vi "HostCurrentSampling.vi"() -> ()   [LabVIEW 2014]
uses:
  <vilib>/FPGAPlugInAG/PCIe-7851R/niLvFpga_Open_PCIe-7851R.vi
  <vilib>/rvi/interface/common/dynamic/niFpgaDynamicAddResources.vi
  <vilib>/Utility/error.llb/Error Cluster From Error Code.vi
  <vilib>/rvi/errors/niLvFpgaAdjustHostInterfaceError.vi
  <vilib>/FPGAPlugInAG/Dynamic/niLvFpga_Close_Dynamic.vi
  <vilib>/rvi/interface/nirviOpenFPGA/nirviOpenFPGA.xnode
  FPGA Bitfiles/UntitledProject1_FPGATarget_FPGACurrentSampl_waaLAvbA01k.lvbitx
  <vilib>/rvi/interface/nirviReadWriteControl/nirviReadWriteControl.xnode
  <vilib>/rvi/interface/nirviMethod/nirviMethod.xnode
  <vilib>/rvi/interface/nirviCloseFPGA/nirviCloseFPGA.xnode
  NiFpgaLv.dll
  <vilib>/rvi/interface/Simulation/niFpgaSimulationCallBeginRW.vi
  <vilib>/FPGAPlugInAG/Dynamic/niLvFpga_ReadFifo_Dynamic.vi
  <vilib>/rvi/errors/niLvFpgaMergeErrorWithErrorCode.vi
panel:
  in  "Count(uSec)":u32
  out "PresNum":i32
  in  "SampleNum":i32
  in  "stop":bool
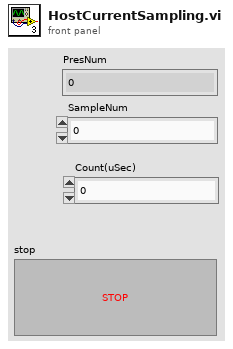
[diagram p1: front panel]
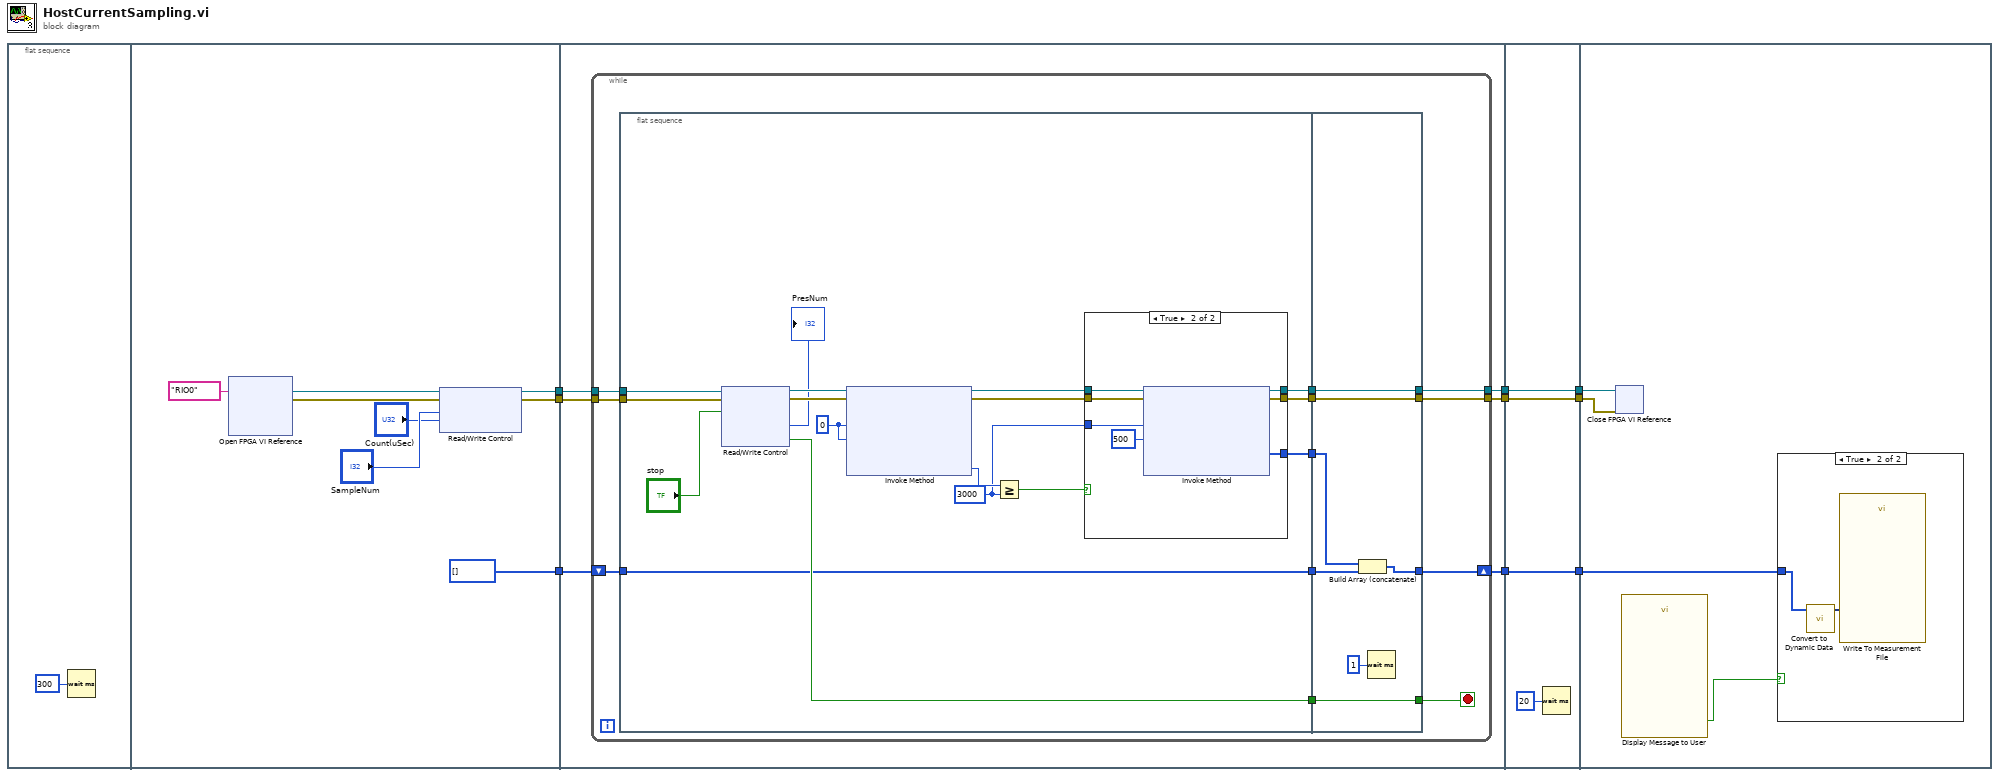
[diagram p0: block diagram]
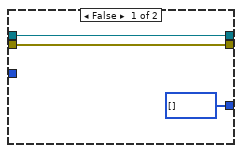
[diagram p2: hidden frame]
diagram:
  n1 = flat-sequence {
    tunnel: [w15] -> w9
    tunnel: [w14] -> w8
    tunnel: [i16[] [] ("Data")] -> w3
    tunnel: w9 -> [w24]
    tunnel: w8 -> [w23]
    tunnel: [w22] -> w7
    tunnel: [w21] -> w6
    tunnel: w3 -> [w20]
    tunnel: [w19] -> w2
    tunnel: w7 -> [w73]
    tunnel: w6 -> [w72]
    tunnel: [w73] -> w5
    tunnel: [w72] -> w4
    tunnel: w2 -> [w71]
    tunnel: [w71] -> w1
    tunnel: w5 -> [w78]
    tunnel: w4 -> [w77]
    tunnel: w1 -> [w75]
    frame #0 {
      n2 = Wait (ms)(milliseconds to wait=u32 300) -> ()  [unwired: 1 out]
    }
    frame #1 {
      n3 = xnode "Open FPGA VI Reference"("resource name"=tag "RIO0") -> ("FPGA VI Reference Out"=w17:refnum<k20>, "error out"=w16:errorcluster)  [unwired: 1 in]
      n4 = xnode "Read/Write Control"("FPGA VI Reference In"=w17, "error in"=w16, "SampleNum"="SampleNum", "Count(uSec)"="Count(uSec)") -> ("FPGA VI Reference Out"=w15:refnum<k20>, "error out"=w14:errorcluster)
    }
    frame #2 {
      n5 = while {
        tunnel: w24 -> [w36]
        tunnel: w23 -> [w35]
        tunnel: [w34] -> w22
        tunnel: [w33] -> w21
        shift-right: [w26] -> w19
        shift-left: w20 -> [w27]
        stop <- w29 stop-if-true
        n6 = flat-sequence {
          tunnel: w36 -> [w53]
          tunnel: w35 -> [w52]
          tunnel: [w42] -> w32
          tunnel: [w41] -> w31
          tunnel: [w50] -> w30
          tunnel: [w38] -> w28
          tunnel: w27 -> [w37]
          tunnel: [w37] -> w25
          tunnel: [w69] -> w33
          tunnel: [w70] -> w34
          tunnel: [w68] -> w29
          tunnel: w30 -> [w68]
          tunnel: w31 -> [w69]
          tunnel: w32 -> [w70]
          tunnel: w28 -> [w66]
          tunnel: [w64] -> w26
          tunnel: w25 -> [w65]
          frame #0 {
            w39 = u32 3000 ("y")
            w47 = u32 0 ("Number of Elements")
            n7 = xnode "Read/Write Control"("FPGA VI Reference In"=w53, "error in"=w52, "stop"="stop") -> ("FPGA VI Reference Out"=w49:refnum<k20>, "error out"=w48:errorcluster, "PresNum"=→"PresNum":i32, "Stopped?"=w50:bool)
            n8 = xnode "Invoke Method"("FPGA VI Reference In"=w49, "error in"=w48, "Number of Elements"=w47, "Timeout (ms)"=w47) -> ("FPGA VI Reference Out"=w46:refnum<k20>, "error out"=w45:errorcluster, "Elements Remaining"=w44:u32)  [unwired: 1 out]
            n9 = Greater Or Equal?(x=w44, y=w39) -> (x >= y?=w43:bool)
            n10 = case shown="True" w43 {
              tunnel: w46 -> [w56 w63]
              tunnel: w45 -> [w55 w62]
              tunnel: [w56 w61] -> w42
              tunnel: [w55 w60] -> w41
              tunnel: w39 -> [_ w59]
              tunnel: [i16[] [] ("Data") w57] -> w38
              frame False {
              }
              frame True {
                n11 = xnode "Invoke Method"("FPGA VI Reference In"=w63, "error in"=w62, "Number of Elements"=w59, "Timeout (ms)"=500) -> ("FPGA VI Reference Out"=w61:refnum<k20>, "error out"=w60:errorcluster, "Data"=w57:i16[])  [unwired: 1 out]
              }
            }
          }
          frame #1 {
            n12 = Build Array (concatenate)(w66, w65) -> (w64:i16[])
            n13 = Wait (ms)(milliseconds to wait=u32 1) -> ()  [unwired: 1 out]
          }
        }
      }
    }
    frame #3 {
      n14 = Wait (ms)(milliseconds to wait=u32 20) -> ()  [unwired: 1 out]
    }
    frame #4 {
      n15 = xnode "Close FPGA VI Reference"("FPGA VI Reference In"=w78, "error in"=w77) -> ()  [unwired: 1 out]
      n16 = call "Display Message to User"() -> ("OK"=w76:bool)  [unwired: 10 in, 1 out]
      n17 = case shown="True" w76 {
        tunnel: w75 -> [_ w80]
        frame False {
        }
        frame True {
          n18 = call "Convert to Dynamic Data"("Array"=w80) -> ("Dynamic Data Type"=w79:dynamicdata)  [unwired: 3 in]
          n19 = call "Write To Measurement File"("Signals"=w79) -> ()  [unwired: 16 in, 3 out]
        }
      }
    }
  }
